vi "LIndex.vi"(0 "reference in":refnum<class "Redis.lvclass">, 1 "Key":string, 7 "Index":u32, 11 "Error In":errorcluster) -> (4 "reference out":refnum<class "Redis.lvclass">, 8 "Value":string, 15 "Error Out":errorcluster)   [LabVIEW 2020, in "Redis.lvclass"]
doc: "<b>LINDEX</b>\n\nReturns the element at index index in the list stored at key. The index is zero-based, so 0 means the first element, 1 the second element and so on. Negative indices can be used to designate elements starting at the tail of the list. Here, -1 means the last element, -2 means the penultimate and so forth."
uses:
  Redis.lvclass
  Redis.lvclass/Redis.ctl
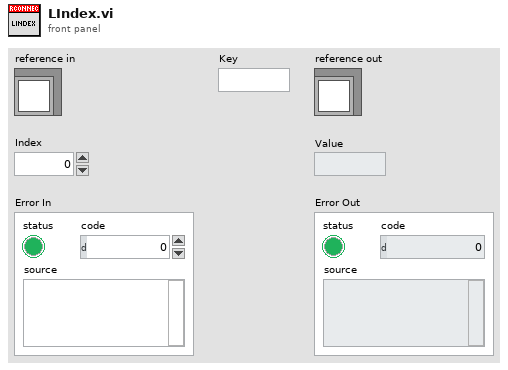
[diagram p1: front panel]
types:
  T1 = typedef "Redis.lvclass/RedisDataType.ctl" = cluster{"Reply Type":T2, "Integer":i64, "String":string, "Multibulk":variant[], "StringData":string[]}
  T2 = typedef "Redis.lvclass/ReplyDataTypeEnum.ctl" = enum16{"None", "Error", "Status", "Nil", "Integer", "String", "Multibulk"}
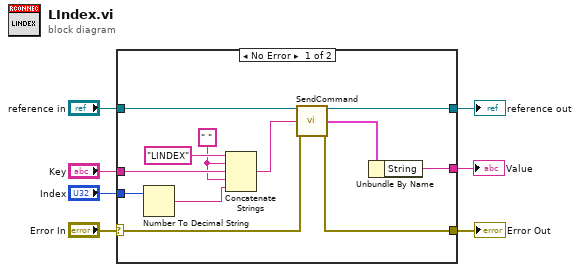
[diagram p0: block diagram]
diagram:
  n1 = case shown="No Error" "Error In" {
    selector: "Error In" -> [w17 w21]
    tunnel: [w16 w21] -> w6
    tunnel: [w19 w20] -> w4
    tunnel: "reference in" -> [w18 w20]
    tunnel: "Key" -> [w14 _]
    tunnel: "Index" -> [w11 _]
    tunnel: [w8 _] -> w1
    frame No Error {
      w12 = " "
      n2 = Number To Decimal String(number=w11) -> (decimal integer string=w10:string)  [unwired: 1 in]
      n3 = Concatenate Strings("LINDEX", w12, w14, w12, w10) -> (w13:string)
      n4 = call "SendCommand.vi"("reference in"=w18, "Command"=w13, "Error In"=w17) -> ("reference out"=w19:refnum<class "Redis.lvclass">, "Data"=w9:T1, "Error Out"=w16:errorcluster)  [unwired: 10 in]
      n5 = Unbundle By Name(w9) -> ("String"=w8:string)
    }
    frame Error {
    }
  }
  "Error Out" <- w6
  "reference out" <- w4
  "Value" <- w1
